vi "Read Waveform.vi"(8 "error in (no error)":errorcluster, 9 "Source (0: Channel 1)":u16(ring) items=["Channel 1", "Channel 2", "Channel 3", "Channel 4", "Math", "Reference A", "Reference B", "Reference C", "Reference D", "FFT"], 10 "Timeout (10000 ms)":u32=10000, 11 "Osciloscope in":refnum<class "Osciloscope.lvclass">) -> (0 "error out":errorcluster, 1 "Waveform Data":waveform(dbl)(graph), 3 "Osciloscope out":refnum<class "Osciloscope.lvclass">)   [LabVIEW 2020, in "Controlador.lvlib" / "Osciloscope.lvclass"]
uses:
  Osciloscope.lvclass
  Osciloscope.lvclass/Osciloscope.ctl
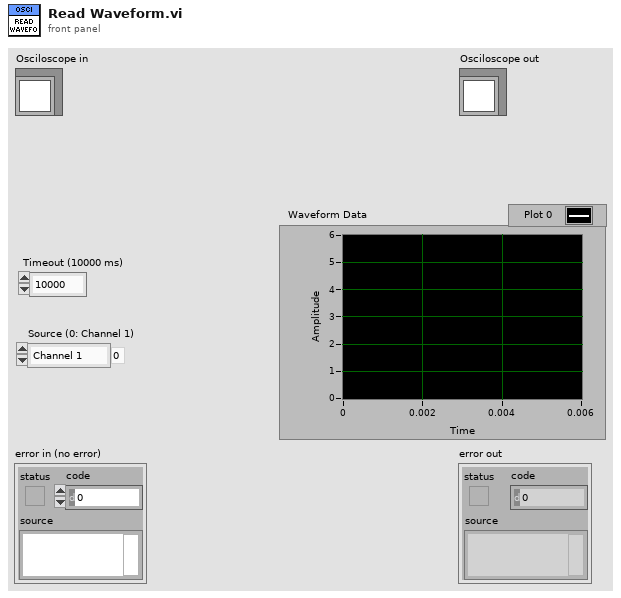
[diagram p1: front panel]
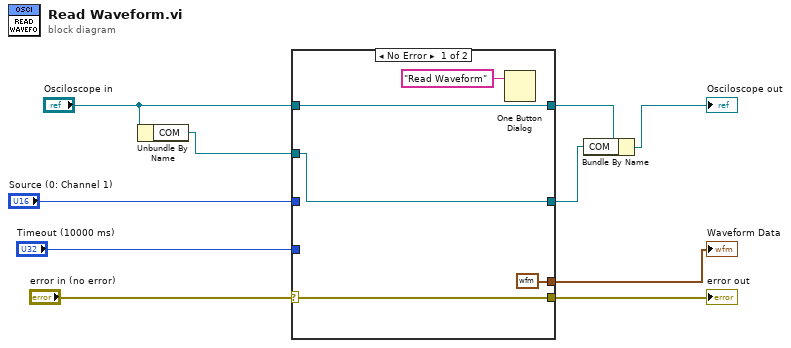
[diagram p0: block diagram]
diagram:
  n1 = Unbundle By Name("Osciloscope in") -> ("COM"=w2:refnum<visa-resource-name>)
  n2 = case shown="No Error" "error in (no error)" {
    selector: "error in (no error)" -> [w14 w17]
    tunnel: [w14 w17] -> w9
    tunnel: [w15 w16] -> w5
    tunnel: "Osciloscope in" -> [w15 w16]
    tunnel: w2 -> [w13 _]
    tunnel: "Source (0: Channel 1)" -> [_ _]
    tunnel: "Timeout (10000 ms)" -> [_ _]
    tunnel: [w13 _] -> w1
    tunnel: [waveform(dbl) {"t0"=timestamp(0 s since 1904-01-01), "dt"=1.0, "Y"=[]} ("Waveform Data") _] -> w6
    frame No Error {
      n3 = One Button Dialog(message="Read Waveform") -> ()  [unwired: 1 in, 1 out]
    }
    frame Error {
    }
  }
  "error out" <- w9
  "Waveform Data" <- w6
  n4 = Bundle By Name(cluster=w5, "COM"=w1) -> (→"Osciloscope out":refnum<class "Osciloscope.lvclass">)
